vi "Query SYMLINK conventions.vi"(11 "session in":refnum<class "Session.lvclass">) -> (1 "OpenSSH?":bool, 2 "detected?":bool, 3 "session out":refnum<class "Session.lvclass">)   [LabVIEW 2020, in "NI_SFTP.lvlib" / "Session.lvclass"]
uses:
  <vilib>/net/SFTP/Session/Session.lvclass
  <vilib>/net/SFTP/Session/Session.lvclass/Session.ctl
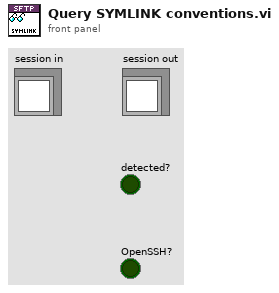
[diagram p1: front panel]
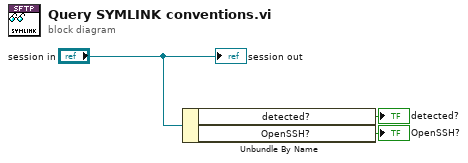
[diagram p0: block diagram]
diagram:
  n1 = Unbundle By Name("session in") -> ("detected?"=→"detected?":bool, "OpenSSH?"=→"OpenSSH?":bool)
  "session out" <- "session in"
